vi "swimbladderControllers_run.vi"(8 "error in (no error)":errorcluster) -> (0 "error out":errorcluster)   [LabVIEW 2013]
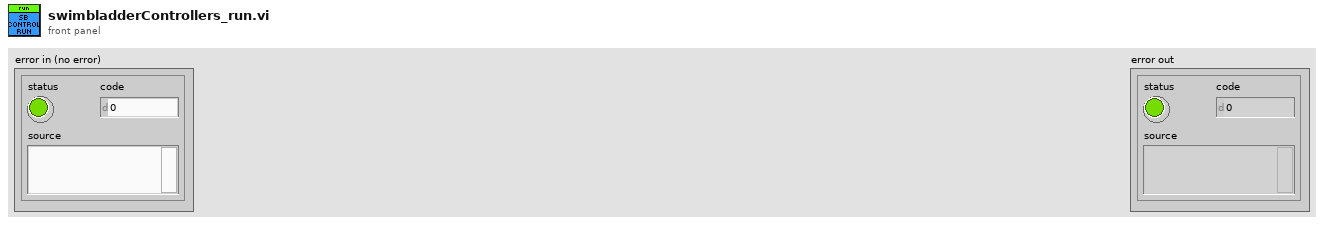
[diagram p1: front panel]
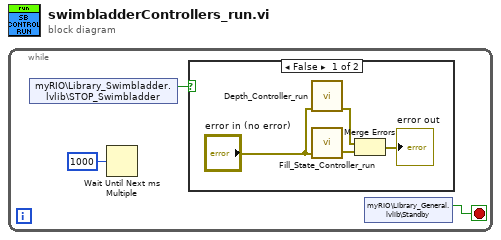
[diagram p0: block diagram]
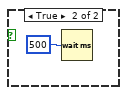
[diagram p2: hidden frame]
diagram:
  n1 = while {
    stop <- w2 stop-if-true
    n2 = shared-variable "myRIO\\Library_Swimbladder.lvlib\\STOP_Swimbladder"() -> (w3:bool)  [unwired: 1 in, 1 out]
    n3 = Wait Until Next ms Multiple(millisecond multiple=u32 1000) -> ()  [unwired: 1 out]
    n4 = case shown="False" w3 {
      frame False {
        n5 = call "Depth_Controller_run.vi"("error in (no error)"="error in (no error)") -> ("error out"=w6:errorcluster)  [unwired: 10 in]
        n6 = call "Fill_State_Controller_run.vi"("error in (no error)"="error in (no error)") -> ("error out"=w5:errorcluster)  [unwired: 3 in]
        n7 = Merge Errors(w6, w5) -> (→"error out":errorcluster)
      }
      frame True {
        n8 = Wait (ms)(milliseconds to wait=u32 500) -> ()  [unwired: 1 out]
      }
    }
    n9 = shared-variable "myRIO\\Library_General.lvlib\\Standby"() -> (w2:bool)  [unwired: 1 in, 1 out]
  }
